vi "serial_mvmnt_terMINATE.vi"(1 "error in":errorcluster) -> (0 "error out":errorcluster)   [LabVIEW 2016]
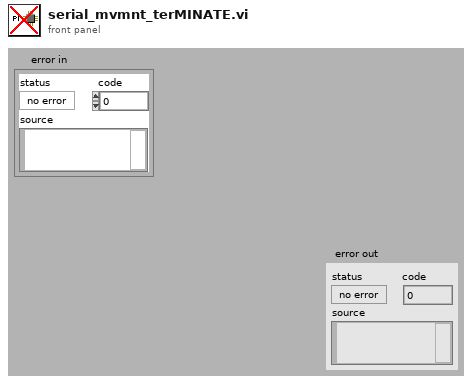
[diagram p1: front panel]
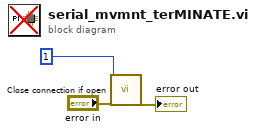
[diagram p0: block diagram]
diagram:
  n1 = call "Close connection if open.vi"("System no."=1, "error in"="error in") -> ("error out"=→"error out":errorcluster)  [unwired: 1 in, 16 out]
